vi "MockInclin.vi"(11 "MockInclinSettings":T1={"ModbusRxDataFIFO"="ModbusInclinRxDataFIFO", "ModbusTxDataFIFO"="ModbusInclinTxDataFIFO", "BufferUpdateFIFO"="MockInclinCommand", "InclinAngleMemory"="MockInlcinAngle"}) -> ()   [LabVIEW 2016, in "FPGAMockInclin.lvlib"]
uses:
  FPGAMockInclin.lvlib
  DataTypes/MockInclinSettings.ctl
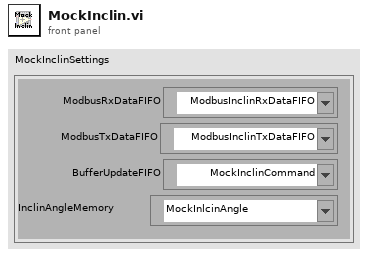
[diagram p1: front panel]
types:
  T1 = typedef "FPGAMockInclin.lvlib/MockInclinSettings.ctl" = cluster{"ModbusRxDataFIFO":refnum<k21>, "ModbusTxDataFIFO":refnum<k21>, "BufferUpdateFIFO":refnum<k21>, "InclinAngleMemory":refnum<k21>}
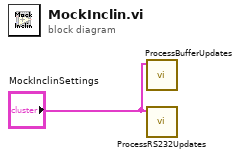
[diagram p0: block diagram]
diagram:
  n1 = call "ProcessBufferUpdates.vi"("MockInclinSettings"="MockInclinSettings") -> ()  [unwired: 11 in]
  n2 = call "ProcessRS232Updates.vi"("MockInclinSettings"="MockInclinSettings") -> ()  [unwired: 11 in]
